vi "Log Message.vi"(8 "error in":errorcluster, 10 "MSG In":string, 11 "session in":T1) -> (0 "error out":errorcluster, 3 "session out":T1)   [LabVIEW 2014, in "System Log.lvclass"]
uses:
  System Log.lvclass
  <userlib>/_Session Fwk/Typedefs/Session Handle.ctl
  <userlib>/_Session Fwk/Session - Root.lvclass
  Controls/DVR.ctl
  System Log.lvclass/System Log.ctl
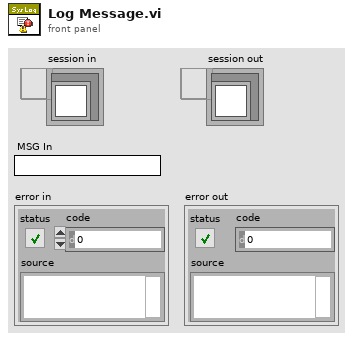
[diagram p1: front panel]
types:
  T1 = typedef "Session - Root.lvclass/Session Handle.ctl" = refnum<data-value>
  T2 = typedef "System Log.lvclass/DVR.ctl" = refnum<data-value>
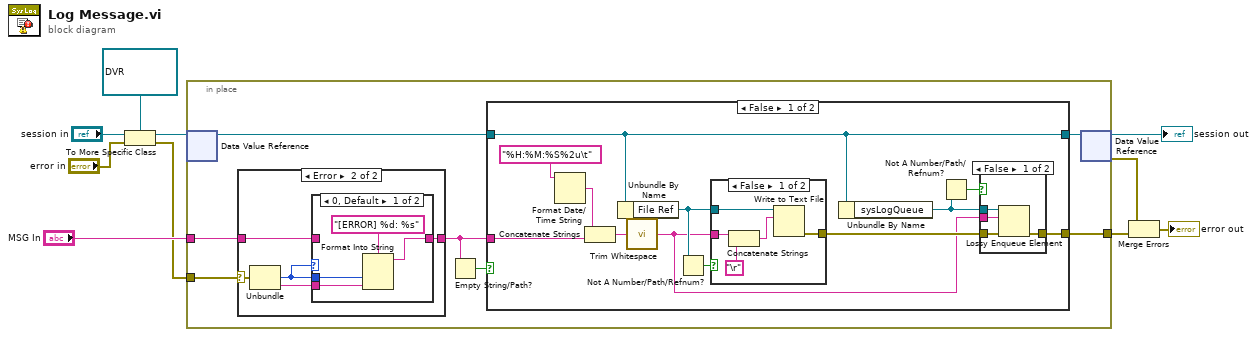
[diagram p0: block diagram]
diagram:
  n1 = To More Specific Class(target class=T2 refnum ("DVR"), reference="session in", error in="error in") -> (specific class reference=w6:T2, error out=w1:errorcluster)
  n2 = in-place {
    in-place-border: w1 -> [w17]
    in-place-border: "MSG In" -> [w16]
    in-place-border: [w11] -> w8
    n3 = in-place-dvr #1(w6) -> (w15:refnum<class "System Log.lvclass">)  [unwired: 1 out]
    n4 = case shown="Error" w17 {
      selector: w17 -> [_ w46]
      tunnel: w16 -> [w41 w42]
      tunnel: [w41 w44] -> w12
      frame No Error {
      }
      frame Error {
        n5 = Unbundle(w46) -> ("code"=w43:i32, "source"=w45:string)  [unwired: 1 out]
        n6 = case shown="0, Default" w43 {
          tunnel: w43 -> [w50 _]
          tunnel: w45 -> [w48 _]
          tunnel: [w47 w51] -> w44
          tunnel: w42 -> [_ w51]
          frame 0, Default {
            n7 = Format Into String(format string="[ERROR] %d: %s", w50, w48) -> (resulting string=w47:string)  [unwired: 2 in, 1 out]
          }
          frame -1073807339 {
          }
        }
      }
    }
    n8 = Empty String/Path?(string/path=w12) -> (empty?=w14:bool)
    n9 = case shown="False" w14 {
      tunnel: w15 -> [w27 w40]
      tunnel: [w27 w40] -> w13
      tunnel: w12 -> [w20 _]
      tunnel: [w25 _] -> w11
      frame False {
        n10 = Format Date/Time String(time format string (%c)="%H:%M:%S%2u\t") -> (date/time string=w21:string)  [unwired: 2 in]
        n11 = Concatenate Strings(w21, w20) -> (w19:string)
        n12 = Unbundle By Name(w27) -> ("File Ref"=w29:refnum<file>)
        n13 = call <vilib>:"Trim Whitespace.vi"("string"=w19) -> ("trimmed string"=w18:string)  [unwired: 1 in]
        n14 = Not A Number/Path/Refnum?(number/path/refnum=w29) -> (NaN/Path/Refnum?=w28:bool)
        n15 = case shown="False" w28 {
          tunnel: w29 -> [w39 _]
          tunnel: w18 -> [w37 _]
          tunnel: [w38 _] -> w26
          frame False {
            n16 = Concatenate Strings(w37, "\r") -> (w35:string)
            n17 = Write to Text File(file (use dialog)=w39, text=w35) -> (error out=w38:errorcluster)  [unwired: 2 in, 2 out]
          }
          frame True {
          }
        }
        n18 = Unbundle By Name(w27) -> ("sysLogQueue"=w24:refnum<queue>)
        n19 = Not A Number/Path/Refnum?(number/path/refnum=w24) -> (NaN/Path/Refnum?=w23:bool)
        n20 = case shown="False" w23 {
          tunnel: w18 -> [w33 _]
          tunnel: w26 -> [w32 w34]
          tunnel: [w31 w34] -> w25
          tunnel: w24 -> [w30 _]
          frame False {
            n21 = Lossy Enqueue Element(queue=w30, element=w33, error in (no error)=w32) -> (error out=w31:errorcluster)  [unwired: 3 out]
          }
          frame True {
          }
        }
      }
      frame True {
      }
    }
    n22 = in-place-dvr #1(w13) -> (→"session out":T2, w9:errorcluster)
  }
  n23 = Merge Errors(w9, w8) -> (→"error out":errorcluster)
